vi "FXP_To_Decimal.vi"() -> ()   [LabVIEW 2018]
panel:
  out "x*y":dbl
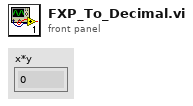
[diagram p1: front panel]
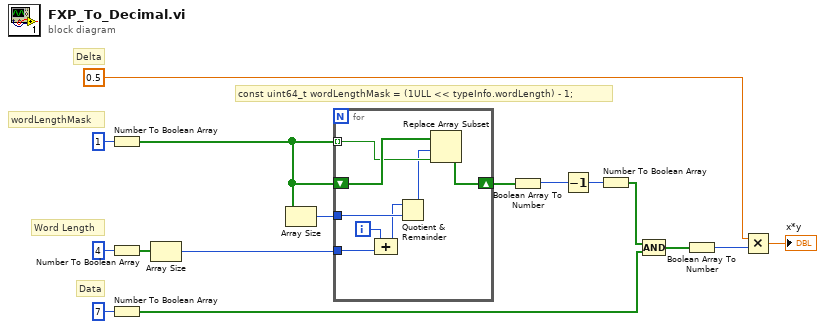
[diagram p0: block diagram]
diagram:
  # "Word Length"
  # "Data"
  # "wordLengthMask"
  # "const uint64_t wordLengthMask = (1ULL << typeInfo.wordLength) - 1;"
  # "Delta"
  n1 = Number To Boolean Array(number=u64 1) -> (Boolean array=w15:bool[])
  n2 = Number To Boolean Array(number=u8 4) -> (Boolean array=w11:bool[])
  n3 = Number To Boolean Array(number=u8 7) -> (Boolean array=w5:bool[])
  n4 = Array Size(array=w11) -> (size(s)=w12:i32)
  n5 = Array Size(array=w15) -> (size(s)=w16:i32)
  n6 = for {
    tunnel: w15 -> [w20] mode=indexing
    shift-right: [w18] -> w10
    shift-left: w15 -> [w21]
    tunnel: w16 -> [w24]
    tunnel: w12 -> [w17]
    i -> [w23]
    n7 = Compound Arithmetic op=ADD(w23, w17) -> (w22:i32)
    n8 = Quotient & Remainder(x=w22, y=w24) -> (x-y*floor(x/y)=w19:i32)  [unwired: 1 out]
    n9 = Replace Array Subset(array=w21, new element=w20, index=w19) -> (w18:bool[])
  }
  n10 = Boolean Array To Number(Boolean array=w10) -> (number=w9:u32)
  n11 = Decrement(x=w9) -> (x-1=w8:u32)
  n12 = Number To Boolean Array(number=w8) -> (Boolean array=w6:bool[])
  n13 = Compound Arithmetic op=AND(w6, w5) -> (w4:bool[])
  n14 = Boolean Array To Number(Boolean array=w4) -> (number=w3:u32)
  n15 = Multiply(x=0.5, y=w3) -> (x*y=→"x*y":dbl)
